vi "启动测量模式选择对话框.vi"(10 "启动选择":u16(ring) items=["水样测试", "标样核查", "零点核查", "跨度核查", "空白测试", "加标回收", "平行样", "校零", "校标"], 11 "确定":bool) -> (3 "启动选择 2":u16(ring) items=["水样测试", "标样核查", "零点核查", "跨度核查", "空白测试", "加标回收", "平行样", "校零", "校标"])   [LabVIEW 2016, in "斯坦道CODMn.lvlib"]
uses:
  <vilib>/Utility/miscctls.llb/LVPointTypeDef.ctl
panel:
  in  "取消":bool
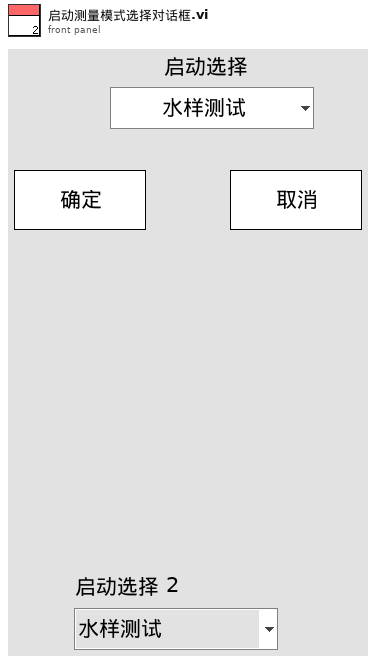
[diagram p1: front panel]
types:
  T1 = typedef "LVPointTypeDef.ctl" = cluster{"Horizontal":i16, "Vertical":i16}
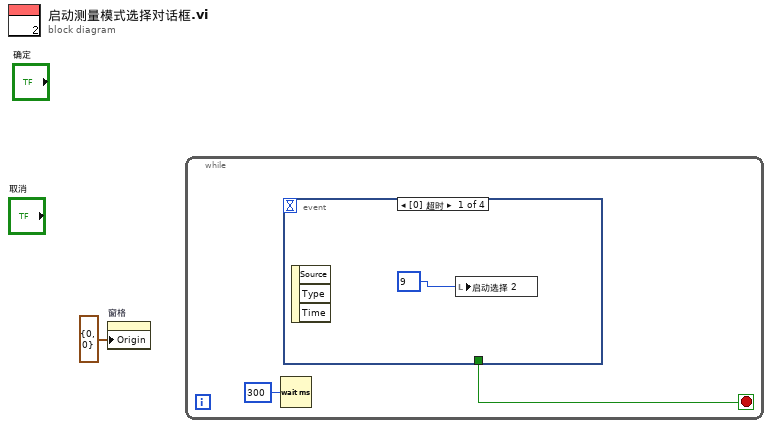
[diagram p0: block diagram]
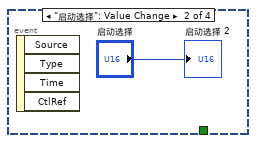
[diagram p2: hidden frame]
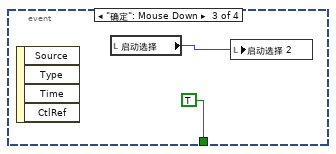
[diagram p3: hidden frame]
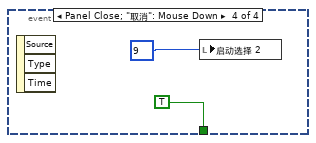
[diagram p4: hidden frame]
diagram:
  n1 = property on="窗格" class="Pane"("Origin"=T1 {"Horizontal"=0, "Vertical"=0} ("原点")) -> ()  [unwired: 2 in, 2 out]
  n2 = while {
    stop <- w3 stop-if-true
    n3 = Wait (ms)(milliseconds to wait=u32 300 ("等待时间（毫秒）")) -> ()  [unwired: 1 out]
    n4 = event shown="[0] 超时" {
      selector: _ -> [_ _ _ _]
      dyn-events: _ -> [_ _ _ _]
      timeout: _ -> [_ _ _ _]
      tunnel: [_ _ TRUE TRUE] -> w3
      event Timeout {
        w4 = u16 9 items=["水样测试", "标样核查", "零点核查", "跨度核查", "空白测试", "加标回收", "平行样", "校零", "校标", ""] ("启动选择 2")
        n5 = event-data() -> ()  [unwired: 1 in, 3 out]
        n6 = local write "启动选择 2"(w4) -> ()
      }
      event "启动选择": Value Change {
        n7 = event-data() -> ()  [unwired: 1 in, 4 out]
        "启动选择 2" <- "启动选择"
      }
      event "确定": Mouse Down {
        n8 = event-data() -> ()  [unwired: 1 in, 4 out]
        n9 = local read "启动选择"() -> (w6:u16)
        n10 = local write "启动选择 2"(w6) -> ()
      }
      event Panel Close; "取消": Mouse Down {
        w8 = u16 9 items=["水样测试", "标样核查", "零点核查", "跨度核查", "空白测试", "加标回收", "平行样", "校零", "校标", ""] ("启动选择 2")
        n11 = event-data() -> ()  [unwired: 1 in, 3 out]
        n12 = local write "启动选择 2"(w8) -> ()
      }
    }
  }
